vi "Read sgl from Register.vi"(8 "error in (no error)":errorcluster, 10 "Start Register":u16, 11 "Sensor General Class in":refnum<class "Sensor General Class.lvclass">) -> (0 "error out":errorcluster, 2 "Data":sgl, 3 "Sensor General Class out":refnum<class "Sensor General Class.lvclass">)   [LabVIEW 2020, in "Sensor General Class.lvclass"]
uses:
  Sensor General Class.lvclass
  Sensor General Class.lvclass/Sensor General Class.ctl
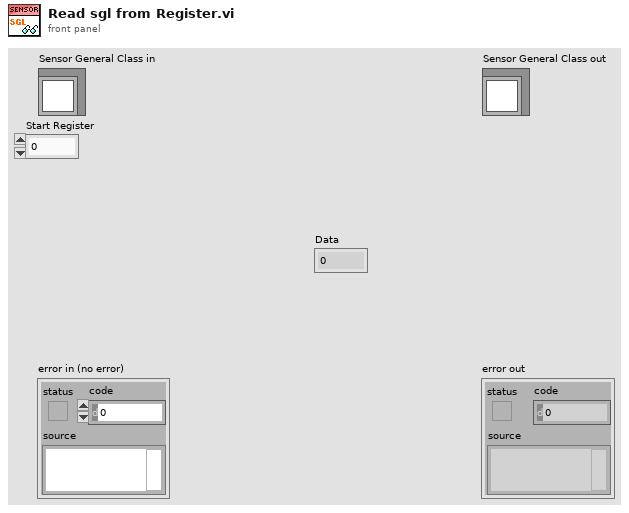
[diagram p1: front panel]
types:
  T1 = cluster{"Mode":enum16{"RTU", "ASCII"}, "Slave Address":u8}
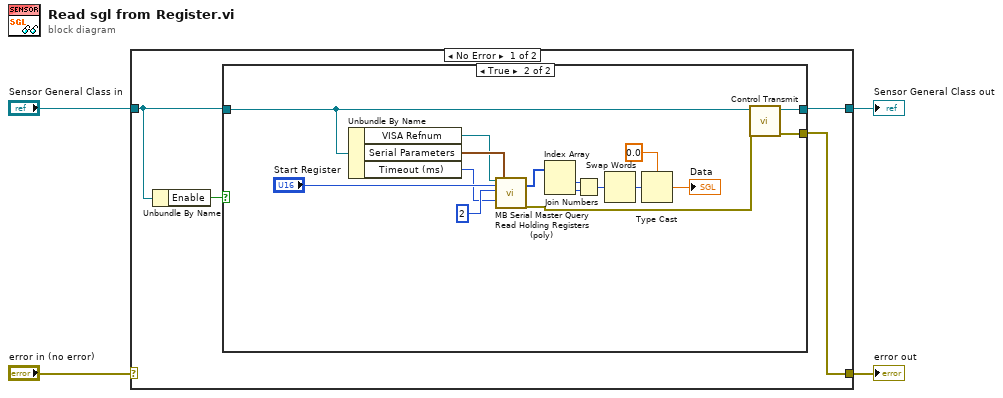
[diagram p0: block diagram]
diagram:
  n1 = case shown="No Error" "error in (no error)" {
    selector: "error in (no error)" -> [_ w27]
    tunnel: [w7 w27] -> w3
    tunnel: [w8 w26] -> w1
    tunnel: "Sensor General Class in" -> [w6 w26]
    frame No Error {
      n2 = Unbundle By Name(w6) -> ("Enable"=w5:bool)
      n3 = case shown="True" w5 {
        tunnel: w6 -> [w9 w13]
        tunnel: [w9 w12] -> w8
        tunnel: [_ w10] -> w7
        frame False {
        }
        frame True {
          n4 = Unbundle By Name(w13) -> ("VISA Refnum"=w23:refnum<visa-resource-name>, "Serial Parameters"=w24:T1, "Timeout (ms)"=w14:u32)
          n5 = call <vilib>:"MB Serial Master Query Read Holding Registers (poly).vi"("VISA resource name"=w23, "Starting Address"="Start Register", "Quantity"=u16 2, "Timeout"=w14, "Serial Parameters"=w24) -> ("Holding Registers"=w18:u16[], "error out"=w11:errorcluster)  [unwired: 11 in, 2 out]
          n6 = Index Array(array=w18) -> (element #1=w20:u16, element #2=w19:u16)  [unwired: 2 in]
          n7 = Join Numbers(hi=w20, lo=w19) -> ((hi.lo)=w22:u32)
          n8 = Swap Words(1:w22) -> (0:w21:u32)
          n9 = Type Cast(type=sgl 0.0 ("p_atm"), x=w21) -> (*(type *) &x=→"Data":sgl)
          n10 = call-dynamic "Control Transmit.vi"("error in (no error)"=w11, "Sensor General Class in"=w13) -> ("error out"=w10:errorcluster, "Sensor General Class out"=w12:refnum<class "Sensor General Class.lvclass">)  [unwired: 8 in]
        }
      }
    }
    frame Error {
    }
  }
  "error out" <- w3
  "Sensor General Class out" <- w1
